vi "SaveConfig.vi"(8 "error in (no error)":errorcluster, 11 "GRMActor in":refnum<class "QuickNoteUI.lvclass">) -> (0 "error out":errorcluster, 3 "GRMActor out":refnum<class "QuickNoteUI.lvclass">)   [LabVIEW 2020, in "QuickNoteUI.lvlib" / "QuickNoteUI.lvclass"]
uses:
  QuickNoteUI.lvclass
  QuickNoteUI.lvclass/QuickNoteUI.ctl
  Hardware Abstraction Layer/Component/GenericActor/GenericActor/GenericController.lvclass
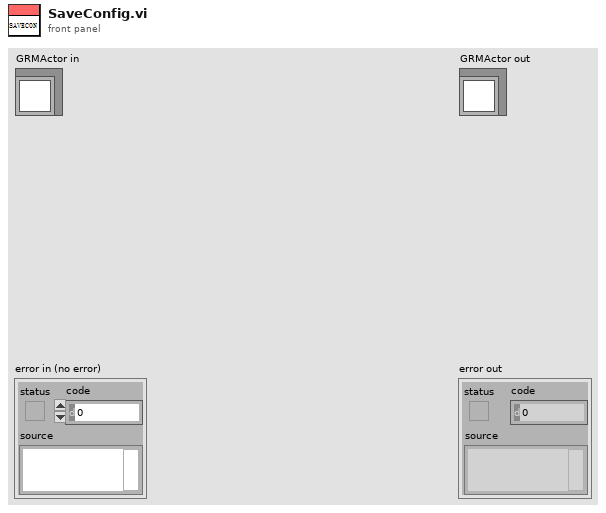
[diagram p1: front panel]
types:
  T1 = typedef "NI_LVConfig.lvlib/Config Data RefNum.ctl" = refnum<k1>
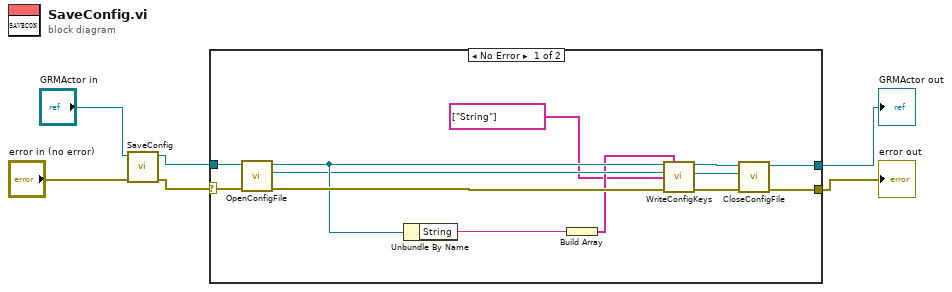
[diagram p0: block diagram]
diagram:
  n1 = call-parent "SaveConfig.vi"("error in (no error)"="error in (no error)", "GRMActor in"="GRMActor in") -> ("error out"=w4:errorcluster, "GRMActor out"=w3:refnum<class "QuickNoteUI.lvclass">)  [unwired: 8 in]
  n2 = case shown="No Error" w4 {
    selector: w4 -> [w19 w20]
    tunnel: [w15 w20] -> w1
    tunnel: [w13 w21] -> w2
    tunnel: w3 -> [w12 w21]
    frame No Error {
      n3 = call-dynamic "OpenConfigFile.vi"("error in (no error)"=w19, "GRMActor in"=w12) -> ("error out"=w16:errorcluster, "refnum"=w10:T1, "GRMActor out"=w11:refnum<class "QuickNoteUI.lvclass">)  [unwired: 7 in]
      n4 = Unbundle By Name(w11) -> ("String"=w17:string)
      n5 = Build Array(w17) -> (w8:string[])
      n6 = call-dynamic "WriteConfigKeys.vi"("GRMActor in"=w11, "StringValues"=w8, "Config Refnum"=w10, "Keys"=string[] ["String"], "error in (no error)"=w16) -> ("GRMActor out"=w14:refnum<class "QuickNoteUI.lvclass">, "Config Refnum dup"=w9:T1, "error out"=w18:errorcluster)  [unwired: 8 in]
      n7 = call-dynamic "CloseConfigFile.vi"("error in (no error)"=w18, "refnum"=w9, "GRMActor in"=w14) -> ("error out"=w15:errorcluster, "GRMActor out"=w13:refnum<class "QuickNoteUI.lvclass">)  [unwired: 7 in]
    }
    frame Error {
    }
  }
  "error out" <- w1
  "GRMActor out" <- w2
